vi "Fast HoloX SLM.vi"   [LabVIEW 2014]
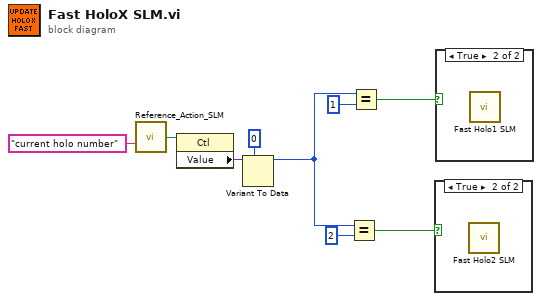
[diagram p0: block diagram]
diagram:
  n1 = call "Reference_Action_SLM.vi"("Control Name"="current holo number") -> ("Ref OUT"=w4:refnum<vi>)  [unwired: 12 in, 2 out]
  n2 = property class="Ctl"(reference=w4) -> ("Value"=w5:variant)  [unwired: 1 in, 2 out]
  n3 = Variant To Data(type=0, Variant=w5) -> (data=w1:i32)  [unwired: 1 in, 1 out]
  n4 = Equal?(x=w1, y=2) -> (x = y?=w6:bool)
  n5 = Equal?(x=w1, y=1) -> (x = y?=w8:bool)
  n6 = case shown="True" w6 {
    frame False {
    }
    frame True {
      n7 = call "Fast Holo2 SLM.vi"() -> ()  [unwired: 12 in]
    }
  }
  n8 = case shown="True" w8 {
    frame False {
    }
    frame True {
      n9 = call "Fast Holo1 SLM.vi"() -> ()  [unwired: 12 in]
    }
  }
